vi "Correct Background File.vi"() -> ()   [LabVIEW 2016]
panel:
  in  "New Background file":path
  in  "Intersept 2":dbl
  in  "Intersept":dbl
  in  "Stop":i32
  in  "Start":i32
  out "Waveform Graph 3":dbl[][](graph)
  out "Waveform Graph 2":dbl[](graph)
  in  "Spectrum file":path
  out "Waveform Graph":dbl[](graph)
  in  "Channel":string="Avg Amplitude"
  in  "Group":string="Raw"
  in  "Background file":path
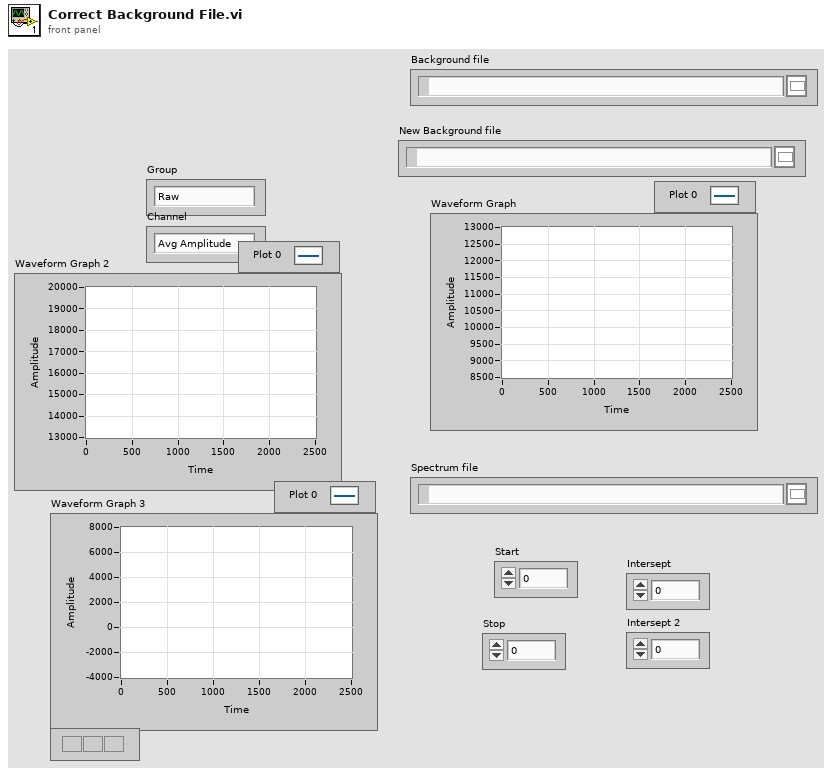
[diagram p1: front panel]
types:
  T1 = enum16{"open", "open or create", "create or replace", "create", "open (read-only)"}
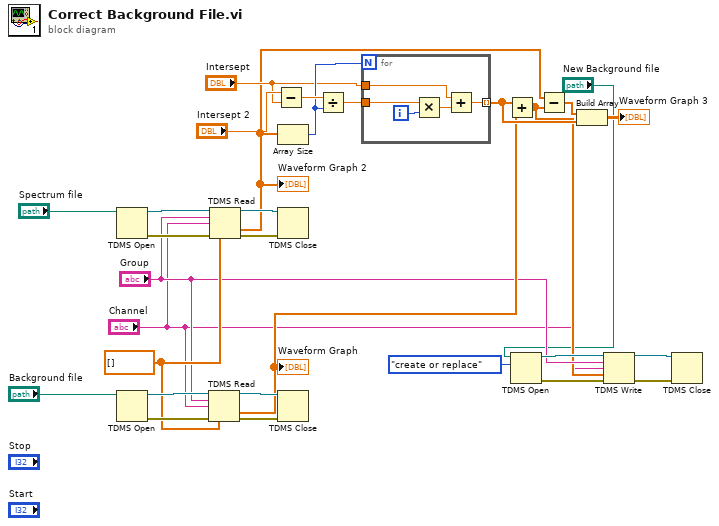
[diagram p0: block diagram]
diagram:
  w11 = dbl[] []
  n1 = TDMS Open(11:"Spectrum file") -> (0:w24:errorcluster, 3:w22:refnum<k34>)  [unwired: 6 in]
  n2 = TDMS Open(11:"Background file") -> (0:w27:errorcluster, 3:w29:refnum<k34>)  [unwired: 6 in]
  n3 = TDMS Read(0:w29, 5:"Group", 7:"Channel", 11:w27, 12:w11) -> (4:w28:refnum<k34>, 10:w12:dbl[], 15:w26:errorcluster)  [unwired: 3 in, 3 out]
  "Waveform Graph" <- w12
  n4 = TDMS Read(0:w22, 5:"Group", 7:"Channel", 11:w24, 12:w11) -> (4:w23:refnum<k34>, 10:w10:dbl[], 15:w25:errorcluster)  [unwired: 3 in, 3 out]
  "Waveform Graph 2" <- w10
  n5 = Subtract(x="Intersept 2", y="Intersept") -> (x-y=w19:dbl)
  n6 = Array Size(array=w10) -> (size(s)=w18:i32)
  n7 = TDMS Close(8:w25, 11:w23) -> ()  [unwired: 2 out]
  n8 = TDMS Close(8:w26, 11:w28) -> ()  [unwired: 2 out]
  n9 = Divide(x=w19, y=w18) -> (x/y=w17:dbl)
  n10 = for {
    N: w18 -> [_]
    tunnel: w17 -> [w35]
    tunnel: "Intersept" -> [w32]
    tunnel: [w31] -> w13 mode=indexing
    i -> [w34]
    n11 = Multiply(x=w35, y=w34) -> (x*y=w33:dbl)
    n12 = Add(x=w32, y=w33) -> (x+y=w31:dbl)
  }
  n13 = Add(x=w13, y=w12) -> (x+y=w4:dbl[])
  n14 = TDMS Open(10:T1."create or replace" ("operation (0:open)"), 11:"New Background file") -> (0:w7:errorcluster, 3:w9:refnum<k34>)  [unwired: 5 in]
  n15 = Subtract(x=w10, y=w4) -> (x-y=w20:dbl[])
  n16 = Build Array(w20, w13) -> (→"Waveform Graph 3":dbl[][])
  n17 = TDMS Write(0:w9, 5:"Group", 7:"Channel", 9:w4, 11:w7) -> (4:w8:refnum<k34>, 15:w6:errorcluster)  [unwired: 1 in, 2 out]
  n18 = TDMS Close(8:w6, 11:w8) -> ()  [unwired: 2 out]
